vi "Color Tables for Displaying the Spectrogram.vi"() -> ()   [LabVIEW 2019]
doc: "This example shows how to apply a customized color table to a spectrogram.\n\n<b>Instructions:</b>\n1) Run this VI.\n2) Change the value of <b>Color Table</b>.\n3) Observe the <b>Spectrogram</b>.\n4) Browse the Block Diagram to learn how to customize a color table to display a spectrogram."
uses:
  <vilib>/addons/Time Frequency Analysis/Spectrogram.llb/TFA STFT Spectrogram (Waveform).vi
  <vilib>/addons/Time Frequency Analysis/_control.llb/TFA Configure Spectrogram Indicator (Predefined Color Table).vi
  <vilib>/addons/Time Frequency Analysis/_control.llb/TFA Configure Spectrogram Indicator (Customized Color Table).vi
  <vilib>/addons/_Advanced Signal Processing/NI_AdvSigProcTFA.lvlib
panel:
  in  "File Path Control":path=path "\\\\eden\\NHMFLDATA/Data/cell3daq/January_2020/012820/p012_012820.tdms"
  in  "Data":u16(ring)=9 items=["PC Fan"=0, "Noisy Chirps"=1, "TDR 1"=2, "TDR 2"=3, "Liquefaction"=4, "Liquefaction Free"=5, "Aneurysm"=6, "Bat"=7, "RF"=8, "Two Gaussian"=9, "Three Gaussian"=10, "Chirp"=11, "Gaussian Chirp"=12, "Cross Chirp"=13, "Doppler"=14, "HOP"=15, "TF Sine"=16, "Three Tone"=17, "Four Tone"=23, "Blood Flow Doppler (phase a)"=20, "Blood Flow Doppler (phase b)"=21, "Heart sound"=22, "Random Noise"=19]
  in  "Color Table":u16(ring) items=["Rainbow", "Inverse gray", "Gray", "Color table 1", "Color table 2", "Color table 3"]
  in  "Stop":bool
  out "aspt-left-top":bool
  out "Spectrogram":dbl[][](graph)
  out "Source Signal":waveform(dbl)(graph)
  # "Overview: Shows how to apply a customized color table to a spectrogram.\nRequirements: LabVIEW Full Development System, Advanced Signal Processing Toolkit\nInstructions: \n1. Run this VI.\n2. Change the value of Color Table.\n3. Observe the Spectrogram.\n4. Browse the block diagram to learn how to customize a color table to display a spectrogram.\n5. Click Stop to stop the VI."
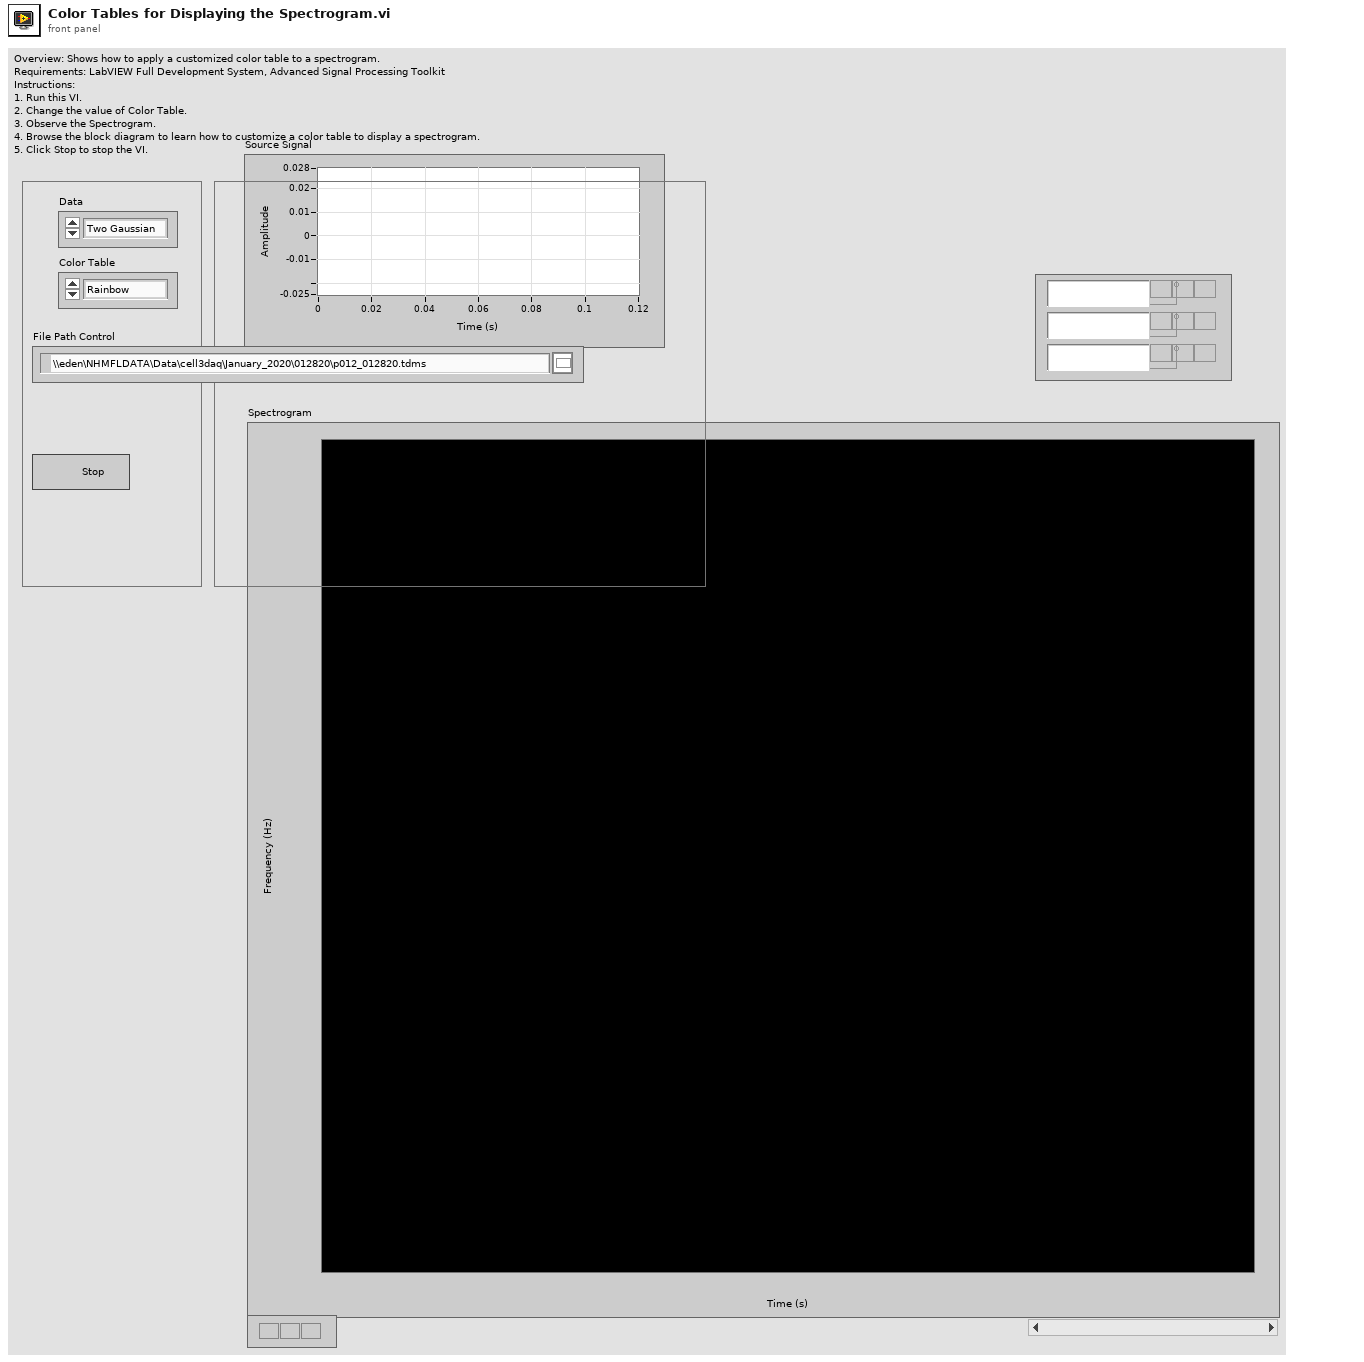
[diagram p1: front panel]
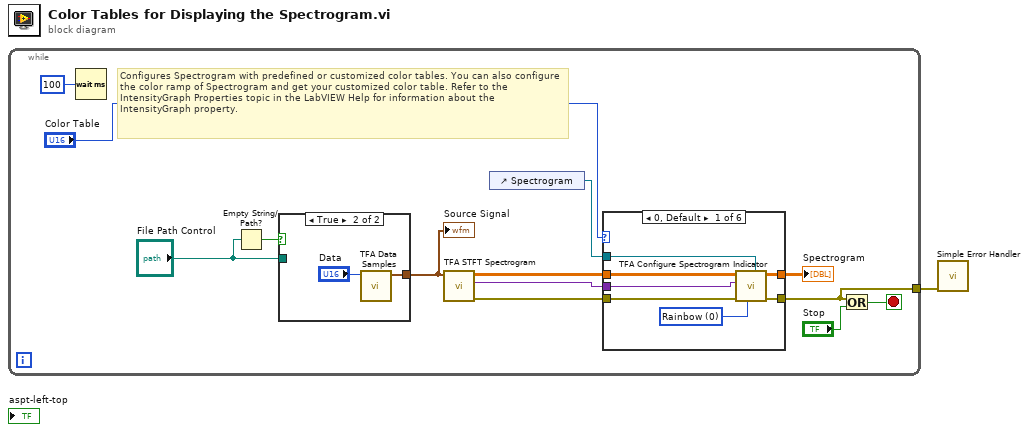
[diagram p0: block diagram]
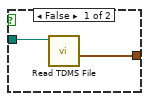
[diagram p2: hidden frame]
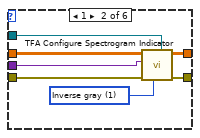
[diagram p3: hidden frame]
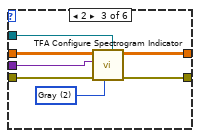
[diagram p4: hidden frame]
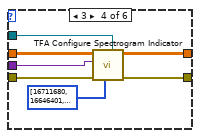
[diagram p5: hidden frame]
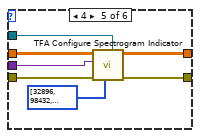
[diagram p6: hidden frame]
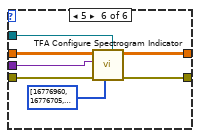
[diagram p7: hidden frame]
diagram:
  n1 = while {
    tunnel: [w5] -> w1
    stop <- w6 stop-if-true
    # "Configures Spectrogram with predefined or customized color tables. You can also configure the color ramp of Spectrogram and get your customized color table. Refer to the IntensityGraph Properties topic in the LabVIEW Help for information about the IntensityGraph property."
    n2 = Wait (ms)(milliseconds to wait=u32 100 ("millisecond multiple")) -> ()  [unwired: 1 out]
    n3 = Empty String/Path?(string/path="File Path Control") -> (empty?=w3:bool)
    n4 = case shown="True" w3 {
      tunnel: [w15 w17] -> w4
      tunnel: "File Path Control" -> [w16 _]
      frame False {
        n5 = call "Read TDMS File.vi"("File Path Control"=w16) -> ("Waveform"=w15:waveform(dbl))  [unwired: 8 in, 2 out]
      }
      frame True {
        n6 = call <vilib>:"TFA Data Samples.vi"("data"="Data") -> ("signal"=w17:waveform(dbl))  [unwired: 10 out]
      }
    }
    "Source Signal" <- w4
    n7 = call-poly <vilib>:"TFA STFT Spectrogram.vi"("signal"=w4) -> ("error out"=w11:errorcluster, "scale info"=w12:variant, "spectrogram"=w13:dbl[][])  [unwired: 3 in, 5 out]
    n8 = control-ref of="Spectrogram"() -> (w8:refnum<vi>)
    n9 = case shown="0, Default" "Color Table" {
      tunnel: w8 -> [w25 w32 w39 w46 w53 w60]
      tunnel: [w24 w31 w38 w45 w52 w59] -> w14
      tunnel: w13 -> [w23 w30 w37 w44 w51 w58]
      tunnel: w12 -> [w22 w29 w36 w43 w50 w57]
      tunnel: w11 -> [w21 w28 w35 w42 w49 w56]
      tunnel: [w19 w26 w33 w40 w47 w54] -> w5
      frame 0, Default {
        w20 = u16 0 items=["Rainbow", "Inverse gray", "Gray"] ("color table")
        n10 = call-poly <vilib>:"TFA Configure Spectrogram Indicator.vi"("reference of TF spectrogram indicator"=w25, "color table"=w20, "error in (no error)"=w21, "scale info"=w22, "spectrogram"=w23) -> ("error out"=w19:errorcluster, "TF spectrogram indicator"=w24:dbl[][])  [unwired: 2 in, 3 out]
      }
      frame 1 {
        w27 = u16 1 items=["Rainbow", "Inverse gray", "Gray"] ("color table")
        n11 = call-poly <vilib>:"TFA Configure Spectrogram Indicator.vi"("reference of TF spectrogram indicator"=w32, "color table"=w27, "error in (no error)"=w28, "scale info"=w29, "spectrogram"=w30) -> ("error out"=w26:errorcluster, "TF spectrogram indicator"=w31:dbl[][])  [unwired: 2 in, 3 out]
      }
      frame 2 {
        w34 = u16 2 items=["Rainbow", "Inverse gray", "Gray"] ("color table")
        n12 = call-poly <vilib>:"TFA Configure Spectrogram Indicator.vi"("reference of TF spectrogram indicator"=w39, "color table"=w34, "error in (no error)"=w35, "scale info"=w36, "spectrogram"=w37) -> ("error out"=w33:errorcluster, "TF spectrogram indicator"=w38:dbl[][])  [unwired: 2 in, 3 out]
      }
      frame 3 {
        n13 = call-poly <vilib>:"TFA Configure Spectrogram Indicator.vi"("reference of TF spectrogram indicator"=w46, "color table"=u32[] [16711680, 16646401, 16581122, 16515843, 16450564, 16385285, 16320006, 16254727, 16189448, 16124169, 16058890, 15993611, 15928332, 15863053, 15797774, 15732495, 15667216, 15601937, 15536658, 15471379, 15406100, 15340821, 15275542, 15210263, 15144984, 15079705, 15014426, 14949147, 14883868, 14818589, 14753310, 14688031, 14622752, 14557473, 14492194, 14426915, 14361636, 14296357, 14231078, 14165799, 14100520, 14035241, 13969962, 13904683, 13839404, 13774125, 13708846, 13643567, 13578288, 13513009, 13447730, 13382451, 13317172, 13251893, 13186614, 13121335, 13056056, 12990777, 12925498, 12860219, 12794940, 12729661, 12664382, 12599103, 12533824, 12468545, 12403266, 12337987, 12272708, 12207429, 12142150, 12076871, 12011592, 11946313, 11881034, 11815755, 11750476, 11685197, 11619918, 11554639, 11489360, 11424081, 11358802, 11293523, 11228244, 11162965, 11097686, 11032407, 10967128, 10901849, 10836570, 10771291, 10706012, 10640733, 10575454, 10510175, 10444896, 10379617, 10314338, 10249059, 10183780, 10118501, 10053222, 9987943, 9922664, 9857385, 9792106, 9726827, 9661548, 9596269, 9530990, 9465711, 9400432, 9335153, 9269874, 9204595, 9139316, 9074037, 9008758, 8943479, 8878200, 8812921, 8747642, 8682363, 8617084, 8551805, 8486526, 8421247, 8355968, 8290689, 8225410, 8160131, 8094852, 8029573, 7964294, 7899015, 7833736, 7768457, 7703178, 7637899, 7572620, 7507341, 7442062, 7376783, 7311504, 7246225, 7180946, 7115667, 7050388, 6985109, 6919830, 6854551, 6789272, 6723993, 6658714, 6593435, 6528156, 6462877, 6397598, 6332319, 6267040, 6201761, 6136482, 6071203, 6005924, 5940645, 5875366, 5810087, 5744808, 5679529, 5614250, 5548971, 5483692, 5418413, 5353134, 5287855, 5222576, 5157297, 5092018, 5026739, 4961460, 4896181, 4830902, 4765623, 4700344, 4635065, 4569786, 4504507, 4439228, 4373949, 4308670, 4243391, 4178112, 4112833, 4047554, 3982275, 3916996, 3851717, 3786438, 3721159, 3655880, 3590601, 3525322, 3460043, 3394764, 3329485, 3264206, 3198927, 3133648, 3068369, 3003090, 2937811, 2872532, 2807253, 2741974, 2676695, 2611416, 2546137, 2480858, 2415579, 2350300, 2285021, 2219742, 2154463, 2089184, 2023905, 1958626, 1893347, 1828068, 1762789, 1697510, 1632231, 1566952, 1501673, 1436394, 1371115, 1305836, 1240557, 1175278, 1109999, 1044720, 979441, 914162, 848883, 783604, 718325, 653046, 587767, 522488, 457209, 391930, 326651, 261372, 196093, 130814, 65535] ("Color Array"), "error in (no error)"=w42, "scale info"=w43, "spectrogram"=w44) -> ("error out"=w40:errorcluster, "TF spectrogram indicator"=w45:dbl[][])  [unwired: 2 in, 3 out]
      }
      frame 4 {
        n14 = call-poly <vilib>:"TFA Configure Spectrogram Indicator.vi"("reference of TF spectrogram indicator"=w53, "color table"=u32[] [32896, 98432, 163968, 229505, 295042, 360578, 426114, 491651, 557188, 622724, 688260, 753797, 819334, 884870, 950406, 1015943, 1081480, 1147016, 1212552, 1278089, 1343626, 1409162, 1474698, 1540235, 1605772, 1671308, 1736844, 1802381, 1867918, 1933454, 1998990, 2064527, 2130064, 2195600, 2261136, 2326673, 2392210, 2457746, 2523282, 2588819, 2654356, 2719892, 2785428, 2850965, 2916502, 2982038, 3047574, 3113111, 3178648, 3244184, 3309720, 3375257, 3440794, 3506330, 3571866, 3637403, 3702940, 3768476, 3834012, 3899549, 3965086, 4030622, 4096158, 4161695, 4227232, 4292768, 4358304, 4423841, 4489378, 4554914, 4620450, 4685987, 4751524, 4817060, 4882596, 4948133, 5013670, 5079206, 5144742, 5210279, 5275816, 5341352, 5406888, 5472425, 5537962, 5603498, 5669034, 5734571, 5800108, 5865644, 5931180, 5996717, 6062254, 6127790, 6193326, 6258863, 6324400, 6389936, 6455472, 6521009, 6586546, 6652082, 6717618, 6783155, 6848692, 6914228, 6979764, 7045301, 7110838, 7176374, 7241910, 7307447, 7372984, 7438520, 7504056, 7569593, 7635130, 7700666, 7766202, 7831739, 7897276, 7962812, 8028348, 8093885, 8159422, 8224958, 8290494, 8356031, 8421568, 8487104, 8552640, 8618177, 8683714, 8749250, 8814786, 8880323, 8945860, 9011396, 9076932, 9142469, 9208006, 9273542, 9339078, 9404615, 9470152, 9535688, 9601224, 9666761, 9732298, 9797834, 9863370, 9928907, 9994444, 10059980, 10125516, 10191053, 10256590, 10322126, 10387662, 10453199, 10518736, 10584272, 10649808, 10715345, 10780882, 10846418, 10911954, 10977491, 11043028, 11108564, 11174100, 11239637, 11305174, 11370710, 11436246, 11501783, 11567320, 11632856, 11698392, 11763929, 11829466, 11895002, 11960538, 12026075, 12091612, 12157148, 12222684, 12288221, 12353758, 12419294, 12484830, 12550367, 12615904, 12681440, 12746976, 12812513, 12878050, 12943586, 13009122, 13074659, 13140196, 13205732, 13271268, 13336805, 13402342, 13467878, 13533414, 13598951, 13664488, 13730024, 13795560, 13861097, 13926634, 13992170, 14057706, 14123243, 14188780, 14254316, 14319852, 14385389, 14450926, 14516462, 14581998, 14647535, 14713072, 14778608, 14844144, 14909681, 14975218, 15040754, 15106290, 15171827, 15237364, 15302900, 15368436, 15433973, 15499510, 15565046, 15630582, 15696119, 15761656, 15827192, 15892728, 15958265, 16023802, 16089338, 16154874, 16220411, 16285948, 16351484, 16417020, 16482557, 16548094, 16613630, 16679166, 16744703] ("Color Array"), "error in (no error)"=w49, "scale info"=w50, "spectrogram"=w51) -> ("error out"=w47:errorcluster, "TF spectrogram indicator"=w52:dbl[][])  [unwired: 2 in, 3 out]
      }
      frame 5 {
        n15 = call-poly <vilib>:"TFA Configure Spectrogram Indicator.vi"("reference of TF spectrogram indicator"=w60, "color table"=u32[] [16776960, 16776705, 16776450, 16776195, 16775940, 16775685, 16775430, 16775175, 16774920, 16774665, 16774410, 16774155, 16773900, 16773645, 16773390, 16773135, 16772880, 16772625, 16772370, 16772115, 16771860, 16771605, 16771350, 16771095, 16770840, 16770585, 16770330, 16770075, 16769820, 16769565, 16769310, 16769055, 16768800, 16768545, 16768290, 16768035, 16767780, 16767525, 16767270, 16767015, 16766760, 16766505, 16766250, 16765995, 16765740, 16765485, 16765230, 16764975, 16764720, 16764465, 16764210, 16763955, 16763700, 16763445, 16763190, 16762935, 16762680, 16762425, 16762170, 16761915, 16761660, 16761405, 16761150, 16760895, 16760640, 16760385, 16760130, 16759875, 16759620, 16759365, 16759110, 16758855, 16758600, 16758345, 16758090, 16757835, 16757580, 16757325, 16757070, 16756815, 16756560, 16756305, 16756050, 16755795, 16755540, 16755285, 16755030, 16754775, 16754520, 16754265, 16754010, 16753755, 16753500, 16753245, 16752990, 16752735, 16752480, 16752225, 16751970, 16751715, 16751460, 16751205, 16750950, 16750695, 16750440, 16750185, 16749930, 16749675, 16749420, 16749165, 16748910, 16748655, 16748400, 16748145, 16747890, 16747635, 16747380, 16747125, 16746870, 16746615, 16746360, 16746105, 16745850, 16745595, 16745340, 16745085, 16744830, 16744575, 16744320, 16744065, 16743810, 16743555, 16743300, 16743045, 16742790, 16742535, 16742280, 16742025, 16741770, 16741515, 16741260, 16741005, 16740750, 16740495, 16740240, 16739985, 16739730, 16739475, 16739220, 16738965, 16738710, 16738455, 16738200, 16737945, 16737690, 16737435, 16737180, 16736925, 16736670, 16736415, 16736160, 16735905, 16735650, 16735395, 16735140, 16734885, 16734630, 16734375, 16734120, 16733865, 16733610, 16733355, 16733100, 16732845, 16732590, 16732335, 16732080, 16731825, 16731570, 16731315, 16731060, 16730805, 16730550, 16730295, 16730040, 16729785, 16729530, 16729275, 16729020, 16728765, 16728510, 16728255, 16728000, 16727745, 16727490, 16727235, 16726980, 16726725, 16726470, 16726215, 16725960, 16725705, 16725450, 16725195, 16724940, 16724685, 16724430, 16724175, 16723920, 16723665, 16723410, 16723155, 16722900, 16722645, 16722390, 16722135, 16721880, 16721625, 16721370, 16721115, 16720860, 16720605, 16720350, 16720095, 16719840, 16719585, 16719330, 16719075, 16718820, 16718565, 16718310, 16718055, 16717800, 16717545, 16717290, 16717035, 16716780, 16716525, 16716270, 16716015, 16715760, 16715505, 16715250, 16714995, 16714740, 16714485, 16714230, 16713975, 16713720, 16713465, 16713210, 16712955, 16712700, 16712445, 16712190, 16711935] ("Color Array"), "error in (no error)"=w56, "scale info"=w57, "spectrogram"=w58) -> ("error out"=w54:errorcluster, "TF spectrogram indicator"=w59:dbl[][])  [unwired: 2 in, 3 out]
      }
    }
    "Spectrogram" <- w14
    n16 = Or(x=w5, y="Stop") -> (x .or. y?=w6:bool)
  }
  n17 = call <vilib>:"Simple Error Handler.vi"("error in (no error)"=w1) -> ()  [unwired: 4 in, 5 out]
